vi "test_Create Data Channel_array type cast.vi"(8 "error in (no error)":errorcluster, 11 "TestCase in":refnum<class "Instrument Addon Scripting API Channels Unit Tests.lvclass">) -> (0 "error out":errorcluster, 3 "TestCase out":refnum<class "Instrument Addon Scripting API Channels Unit Tests.lvclass">)   [LabVIEW 2019, in "Instrument Addon Scripting API Channels Unit Tests.lvclass"]
uses:
  Instrument Addon Scripting API Channels Unit Tests.lvclass
  <vilib>/addons/_JKI Toolkits/VI Tester/TestCase.llb/TestCase.lvclass
  <vilib>/NI/NI VeriStand Advanced SysDef API/SysDef API/Advanced System Definition.lvlib
  <vilib>/NI/NI VeriStand Advanced SysDef API/_SubVIs/SysDef.Search.GUID.vi
  Addon/Addon Shared/SubVIs/Constants.vi
  Addon/Addon Shared/Instrument Addon Shared.lvlib
  APIs/Scripting API/Instrument Addon Scripting API.lvlib
  APIs/Scripting API/TypeDefs/Array Element.ctl
  <vilib>/NI VeriStand/Custom Device API/Custom Device API.lvlib
  Addon/Addon Shared/Types/Type Cast Type.ctl
  Addon/Addon Shared/Types/Endian.ctl
  APIs/Scripting API/TypeDefs/Array Type Cast Settings.ctl
  <vilib>/NI VeriStand/Custom Device API/Get Item Property (U16).vi
  Addon/Addon Shared/Types/Protocol Data Type.ctl
  Addon/Addon Shared/Types/Data Channel Type.ctl
  APIs/Scripting API/Channels/Create Data Channel - Array - Type Cast.vi
  <vilib>/NI/NI VeriStand Advanced SysDef API/_SubVIs/SysDef.Search.GUIDs.vi
  C:/Program Files (x86)/National Instruments/LabVIEW 2019/vi.lib/addons/_JKI Toolkits/VI Tester/TestCase.llb/TestCase.lvclass
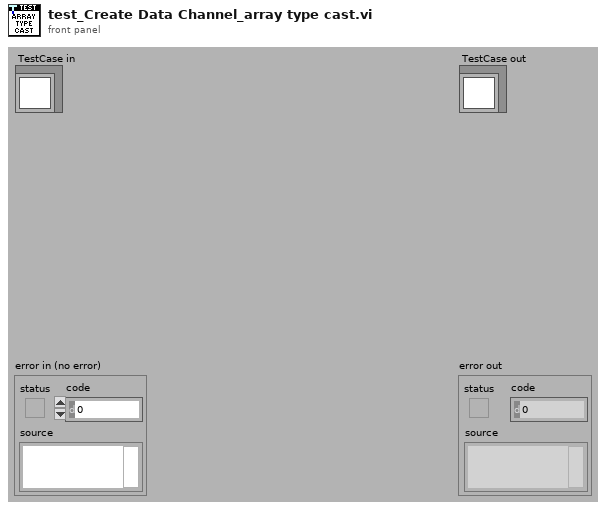
[diagram p1: front panel]
types:
  T1 = typedef "Instrument Addon Scripting API.lvlib/Array Type Cast Settings.ctl" = cluster{"Elements":T2[], "Delimiter":string, "Type":T3, "Endian":T4}
  T2 = typedef "Instrument Addon Scripting API.lvlib/Array Element.ctl" = cluster{"Name":string, "Default Value":dbl, "Units":string}
  T3 = typedef "Instrument Addon Shared.lvlib/Type Cast Type.ctl" = enum16{"DBL", "SGL", "U64", "U32", "U16", "U8", "I64", "I32", "I16", "I8"}
  T4 = typedef "Instrument Addon Shared.lvlib/Endian.ctl" = enum16{"Native", "Little", "Big"}
  T5 = typedef "Instrument Addon Shared.lvlib/Data Channel Type.ctl" = enum16{"Format", "Comparison", "Type Cast", "Enumerated List"}
  T6 = typedef "Instrument Addon Shared.lvlib/Protocol Data Type.ctl" = enum16{"Single Channel", "Array"}
  T7 = typedef "Custom Device API.lvlib/Custom Device Item Ref.ctl" = u64
  T8 = typedef "Advanced System Definition.lvlib/TreeItem.Info.ctl" = cluster{"Name":string, "Description":string, "GUID":string, "Is Channel":bool, "Channel":T9, "Is Waveform":bool, "Waveform":T11}
  T9 = typedef "Custom Device API.lvlib/Custom Device Channel.ctl" = cluster{"Type":T10, "Units":string, "Default Value":dbl, "Faultable":bool, "Scalable":bool}
  T10 = typedef "Custom Device API.lvlib/Custom Device Channel Type.ctl" = enum16{"Input", "Output"}
  T11 = typedef "Custom Device API.lvlib/Custom Device Waveform.ctl" = cluster{"Data Type":T12, "Units":string}
  T12 = typedef "Custom Device API.lvlib/Custom Device Waveform DataType.ctl" = enum16{"Double", "Complex Double"}
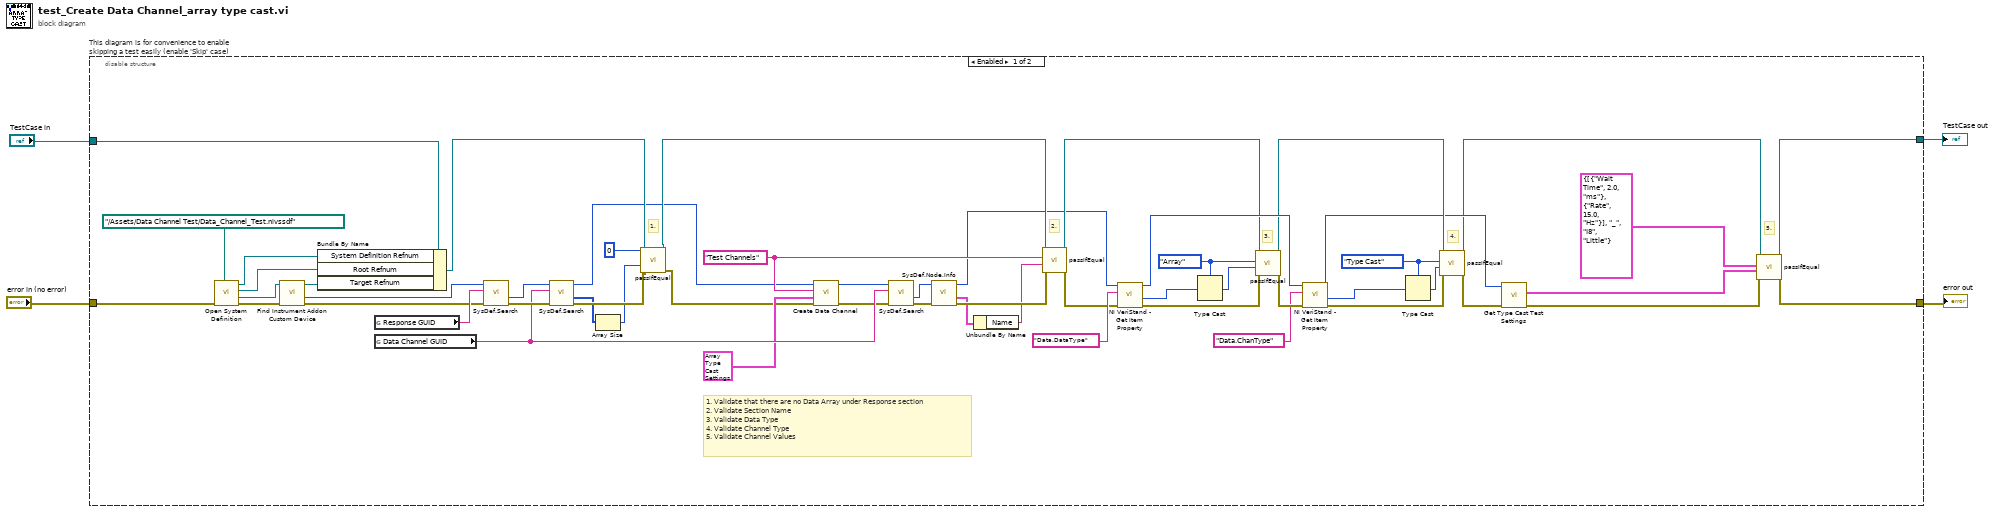
[diagram p0: block diagram]
diagram:
  n1 = disable-structure "This diagram is for convenience to enable skipping a test easily (enable 'Skip' case)" shown="Enabled" {
    disable-tunnel: "TestCase in" -> [w32 w63]
    disable-tunnel: [w36 w61] -> w1
    disable-tunnel: [w37 w62] -> w3
    disable-tunnel: "error in (no error)" -> [w56 w60]
    frame Enabled {
      w16 = Data_Channel_Type."Type Cast" ("Channel Type")
      w21 = Protocol_Data_Type."Array" ("Data Type")
      w45 = "Test Channels" ("Name")
      # "1. Validate that there are no Data Array under Response section\n2. Validate Section Name\n3. Validate Data Type\n4. Validate Channel Type\n5. Validate Channel Values"
      # "4."
      # "3."
      # "5."
      # "2."
      # "1."
      n2 = call "Open System Definition.vi"("error in (no error)"=w56, "System Definition File"=path "../Assets/Data Channel Test/Data_Channel_Test.nivssdf") -> ("error out"=w59:errorcluster, "Target Refnum"=w58:refnum<k24>, "Root Refnum"=w30:refnum<k24>, "System Definition Refnum"=w31:refnum<k24>)  [unwired: 6 in]
      n3 = call "Find Instrument Addon Custom Device.vi"("error in"=w59, "target in"=w58) -> ("error out"=w33:errorcluster, "NodeID"=w55:u64, "target out"=w29:refnum<k24>)  [unwired: 7 in]
      n4 = Bundle By Name(cluster=w32, "System Definition Refnum"=w31, "Root Refnum"=w30, "Target Refnum"=w29) -> (w28:refnum<class "Instrument Addon Scripting API Channels Unit Tests.lvclass">)
      n5 = global read "Constants.vi" "Response GUID"() -> (w54:string)
      n6 = global read "Constants.vi" "Data Channel GUID"() -> (w51:string)
      n7 = call-poly <vilib>:"SysDef.Search.vi"("error in (no error)"=w33, "GUID"=w54, "nodeID"=w55) -> ("error out"=w52:errorcluster, "Value out"=w53:u64)  [unwired: 5 in, 2 out]
      n8 = call-poly <vilib>:"SysDef.Search.vi"("error in (no error)"=w52, "GUID"=w51, "nodeID"=w53) -> ("error out"=w49:errorcluster, "Values Out"=w48:u64[], "nodeID out"=w5:u64)  [unwired: 5 in, 1 out]
      n9 = Array Size(array=w48) -> (size(s)=w47:i32)
      n10 = call-dynamic "passIfEqual.vi"("error in (no error)"=w49, "y"=w47, "x"=0 ("size(s)"), "TestCase in"=w28) -> ("error out"=w27:errorcluster, "TestCase out"=w50:refnum<class "Instrument Addon Scripting API Channels Unit Tests.lvclass">)  [unwired: 6 in]
      n11 = call-poly "Create Data Channel.vi"("error in (no error)"=w27, "settings"=T1 {"Elements"=[{"Name"="Wait Time", "Default Value"=2.0, "Units"="ms"}, {"Name"="Rate", "Default Value"=15.0, "Units"="Hz"}], "Delimiter"="_", "Type"=enum."I8", "Endian"=enum."Little"} ("Settings"), "channel name"=w45, "response refnum in"=w5) -> ("error out"=w44:errorcluster, "response refnum out"=w43:T7)  [unwired: 4 in, 2 out]
      n12 = call-poly <vilib>:"SysDef.Search.vi"("error in (no error)"=w44, "GUID"=w51, "nodeID"=w43) -> ("error out"=w42:errorcluster, "Value out"=w41:u64)  [unwired: 5 in, 2 out]
      n13 = call <vilib>:"SysDef.Node.Info.vi"("error in (no error)"=w42, "nodeID"=w41) -> ("error out"=w40:errorcluster, "Item Info"=w39:T8, "nodeID out"=w10:u64)  [unwired: 6 in, 1 out]
      n14 = Unbundle By Name(w39) -> ("Name"=w38:string)
      n15 = call-dynamic "passIfEqual.vi"("error in (no error)"=w40, "y"=w38, "x"=w45, "TestCase in"=w50) -> ("error out"=w11:errorcluster, "TestCase out"=w12:refnum<class "Instrument Addon Scripting API Channels Unit Tests.lvclass">)  [unwired: 6 in]
      n16 = call-poly <vilib>:"NI VeriStand - Get Item Property.vi"("error in (no error)"=w11, "Property Name"="Data.DataType", "Item Ref in"=w10) -> ("error out"=w24:errorcluster, "Value"=w23:u16, "Item Ref out"=w15:T7)  [unwired: 5 in, 1 out]
      n17 = Type Cast(type=w21, x=w23) -> (*(type *) &x=w22:T6)
      n18 = call-dynamic "passIfEqual.vi"("error in (no error)"=w24, "y"=w22, "x"=w21, "TestCase in"=w12) -> ("error out"=w20:errorcluster, "TestCase out"=w9:refnum<class "Instrument Addon Scripting API Channels Unit Tests.lvclass">)  [unwired: 6 in]
      n19 = call-poly <vilib>:"NI VeriStand - Get Item Property.vi"("error in (no error)"=w20, "Property Name"="Data.ChanType", "Item Ref in"=w15) -> ("error out"=w19:errorcluster, "Value"=w18:u16, "Item Ref out"=w8:T7)  [unwired: 5 in, 1 out]
      n20 = Type Cast(type=w16, x=w18) -> (*(type *) &x=w17:T5)
      n21 = call-dynamic "passIfEqual.vi"("error in (no error)"=w19, "y"=w17, "x"=w16, "TestCase in"=w9) -> ("error out"=w13:errorcluster, "TestCase out"=w7:refnum<class "Instrument Addon Scripting API Channels Unit Tests.lvclass">)  [unwired: 6 in]
      n22 = call "Get Type Cast Test Settings.vi"("Error In"=w13, "Data Channel Ref In"=w8) -> ("Error out"=w35:errorcluster, "Data Channel Settings"=w6:T1)  [unwired: 7 in, 1 out]
      n23 = call-dynamic "passIfEqual.vi"("error in (no error)"=w35, "y"=w6, "x"=T1 {"Elements"=[{"Name"="Wait Time", "Default Value"=2.0, "Units"="ms"}, {"Name"="Rate", "Default Value"=15.0, "Units"="Hz"}], "Delimiter"="_", "Type"=enum."I8", "Endian"=enum."Little"} ("Settings"), "TestCase in"=w7) -> ("error out"=w37:errorcluster, "TestCase out"=w36:refnum<class "Instrument Addon Scripting API Channels Unit Tests.lvclass">)  [unwired: 6 in]
    }
    frame Disabled {
      # "skip test result while test is under development"
      n24 = call <vilib>:"skip.vi"("error in (no error)"=w60, "TestCase in"=w63) -> ("error out"=w62:errorcluster, "TestCase out"=w61:refnum<class "Instrument Addon Scripting API Channels Unit Tests.lvclass">)  [unwired: 8 in]
    }
  }
  "error out" <- w3
  "TestCase out" <- w1
